vi "niRFUtil MT UTIL Buffer block code info.vi"(0 "Symbols In":i32[](array[numeric]) caption="symbols in", 5 "Block Size":i32=1 caption="block size", 11 "error in (no error)":errorcluster, 13 "reset? (T)":bool=TRUE) -> (4 "Symbols Out":i32[](array[numeric]) caption="symbols out", 15 "error out":errorcluster)   [LabVIEW 2015, in "niRFUtil.lvlib"]
uses:
  niRFUtil.lvlib
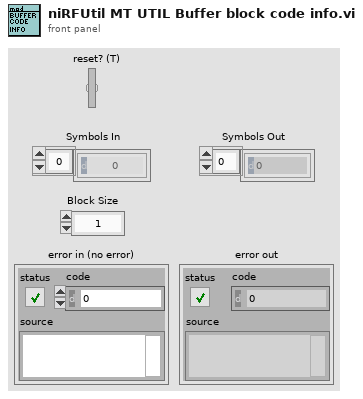
[diagram p1: front panel]
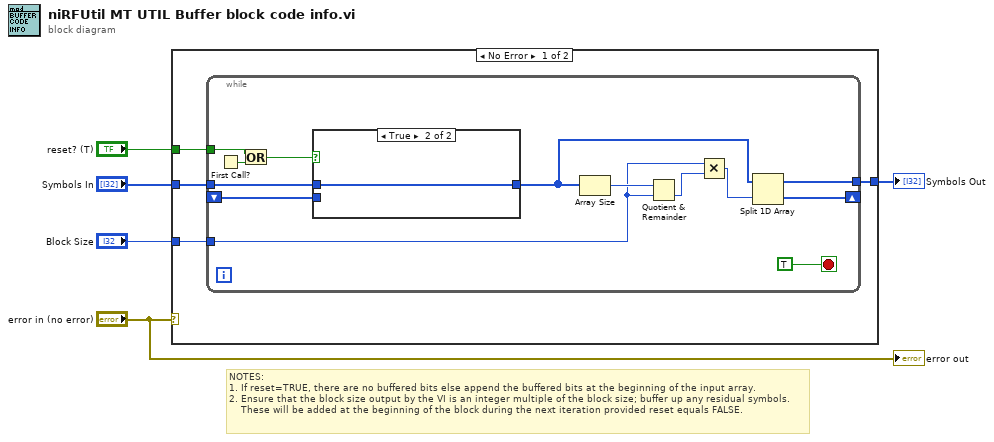
[diagram p0: block diagram]
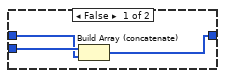
[diagram p2: hidden frame]
diagram:
  # "NOTES:\n1. If reset=TRUE, there are no buffered bits else append the buffered bits at the beginning of the input array.\n2. Ensure that the block size output by the VI is an integer multiple of the block size; buffer up any residual symbols.\n    These will be added at the beginning of the block during the next iteration provided reset equals FALSE."
  n1 = case shown="No Error" "error in (no error)" {
    tunnel: "reset? (T)" -> [w9 _]
    tunnel: "Symbols In" -> [w8 _]
    tunnel: "Block Size" -> [w7 _]
    tunnel: [w6 _] -> w1
    frame No Error {
      n2 = while {
        tunnel: w9 -> [w21]
        tunnel: w8 -> [w18]
        tunnel: w7 -> [w10]
        shift-right: [w13] -> _
        shift-left: _ -> [w12]
        tunnel: [w11] -> w6
        stop <- TRUE stop-if-true
        n3 = First Call?() -> (First Call?: T/F=w20:bool)
        n4 = Or(x=w21, y=w20) -> (x .or. y?=w19:bool)
        n5 = case shown="True" w19 {
          tunnel: w18 -> [w24 w26]
          tunnel: [w23 w26] -> w15
          tunnel: w12 -> [w25 _]
          frame False {
            n6 = Build Array (concatenate)(w25, w24) -> (w23:i32[])
          }
          frame True {
          }
        }
        n7 = Array Size(array=w15) -> (size(s)=w16:i32)
        n8 = Quotient & Remainder(x=w16, y=w10) -> (floor(x/y)=w17:i32)  [unwired: 1 out]
        n9 = Multiply(x=w10, y=w17) -> (x*y=w14:i32)
        n10 = Split 1D Array(array=w15, index=w14) -> (first subarray=w11:i32[], second subarray=w13:i32[])
      }
    }
    frame Error {
    }
  }
  "Symbols Out" <- w1
  "error out" <- "error in (no error)"
